vi "Write Actor Label.vi"(8 "error in":errorcluster, 10 "Actor Label":string, 11 "Monitored Actor in":refnum<class "Monitored Actor.lvclass">) -> (0 "error out":errorcluster, 3 "Monitored Actor out":refnum<class "Monitored Actor.lvclass">)   [LabVIEW 2019, in "Monitored Actor.lvlib" / "Monitored Actor.lvclass"]
doc: "Changes the Actor's Label. This string is displayed in the Actor Monitor window.\n\nPlease see the following web address for additional documentation and tutorial information:\nhttp://www.mooregoodideas.com/monitoring-actors/\n\nAuthor: Derek Trepanier\n\nCopyright (c) 2014, Moore Good Ideas, Inc.\n\nAll rights reserved.\n\nRedistribution and use in source and binary forms, with or without modification, are permitted provided that the following conditions are met:\n\n * Redistributions of source code must retain the above copyright notice, this list of conditions and the following disclaimer.\n * Redistributions in binary form must reproduce the above copyright notice, this list of conditions and the following disclaimer in the documentation and/or other materials provided with the distribution.\n * Neither the name of Moore Good Ideas, Inc. nor the names of its contributors may be used to endorse or promote products derived from this software without specific prior written permission.\n\nTHIS SOFTWARE IS PROVIDED BY THE COPYRIGHT HOLDERS AND CONTRIBUTORS \"AS IS\" AND ANY EXPRESS OR IMPLIED WARRANTIES, INCLUDING, BUT NOT LIMITED TO, THE IMPLIED WARRANTIES OF MERCHANTABILITY AND FITNESS FOR A PARTICULAR PURPOSE ARE DISCLAIMED. IN NO EVENT SHALL THE COPYRIGHT OWNER OR CONTRIBUTORS BE LIABLE FOR ANY DIRECT, INDIRECT, INCIDENTAL, SPECIAL, EXEMPLARY, OR CONSEQUENTIAL DAMAGES (INCLUDING, BUT NOT LIMITED TO, PROCUREMENT OF SUBSTITUTE GOODS OR SERVICES; LOSS OF USE, DATA, OR PROFITS; OR BUSINESS INTERRUPTION) HOWEVER CAUSED AND ON ANY THEORY OF LIABILITY, WHETHER IN CONTRACT, STRICT LIABILITY, OR TORT (INCLUDING NEGLIGENCE OR OTHERWISE) ARISING IN ANY WAY OUT OF THE USE OF THIS SOFTWARE, EVEN IF ADVISED OF THE POSSIBILITY OF SUCH DAMAGE."
uses:
  Monitored Actor.lvclass
  C:/Users/public/Documents/Development/builds/Engine/Actor Framework.lvlibp/1abvi3w/vi.lib/ActorFramework/Actor/Actor.lvclass
  Monitored Actor.lvclass/Monitored Actor.ctl
  Actor Monitor/Actor Monitor Messages/Update Label Msg/Update Label Msg.lvclass
  builds/Engine/Actor Framework.lvlibp/1abvi3w/vi.lib/ActorFramework/Actor/Actor.lvclass
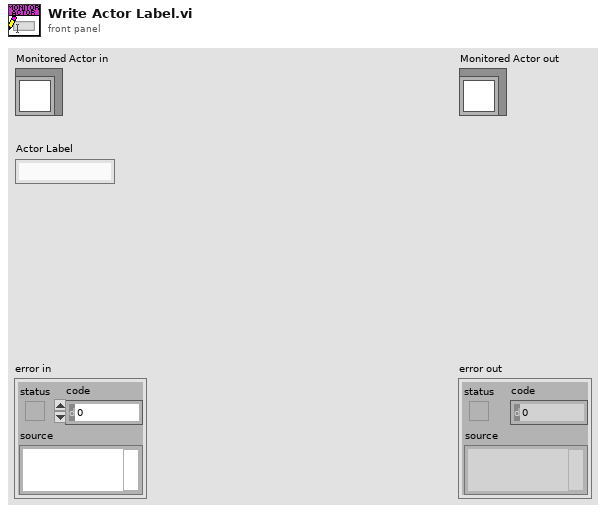
[diagram p1: front panel]
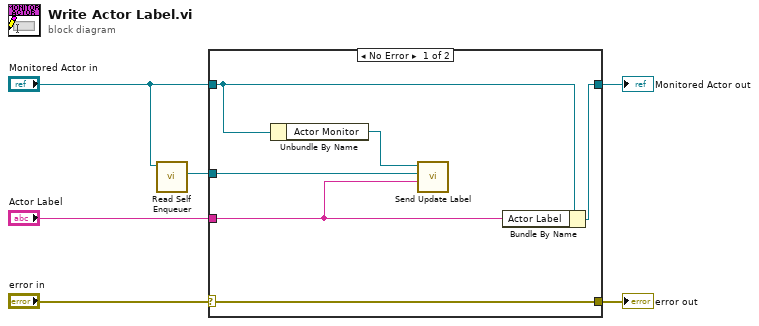
[diagram p0: block diagram]
diagram:
  n1 = call "Read Self Enqueuer.vi"("Actor"="Monitored Actor in") -> ("Self Enqueuer"=w2:refnum<class "Message Enqueuer.lvclass">)  [unwired: 10 in]
  n2 = case shown="No Error" "error in" {
    selector: "error in" -> [w12 w13]
    tunnel: [w12 w13] -> w5
    tunnel: [w11 w14] -> w4
    tunnel: "Monitored Actor in" -> [w10 w14]
    tunnel: "Actor Label" -> [w9 _]
    tunnel: w2 -> [w7 _]
    frame No Error {
      n3 = Unbundle By Name(w10) -> ("Actor Monitor"=w8:refnum<class "Message Enqueuer.lvclass">)
      n4 = call "Send Update Label.vi"("Actor's Label"=w9, "Actor's Self Q"=w7, "Message Enqueuer in"=w8) -> ()  [unwired: 7 in, 2 out]
      n5 = Bundle By Name(cluster=w10, "Actor Label"=w9) -> (w11:refnum<class "Monitored Actor.lvclass">)
    }
    frame Error {
    }
  }
  "error out" <- w5
  "Monitored Actor out" <- w4
